vi "Read Analog Waveforms.vi"(8 "error in":errorcluster, 10 "analog task":refnum<k21>) -> (0 "error out":errorcluster, 2 "analog task out":refnum<k21>, 3 "waveforms":waveform(dbl)[](array[waveform]))   [LabVIEW 2021]
uses:
  <vilib>/DAQmx/read.llb/DAQmx Read (Analog 1D Wfm NChan NSamp).vi
  <vilib>/DAQmx/miscellaneous.llb/DAQmx Fill In Error Info.vi
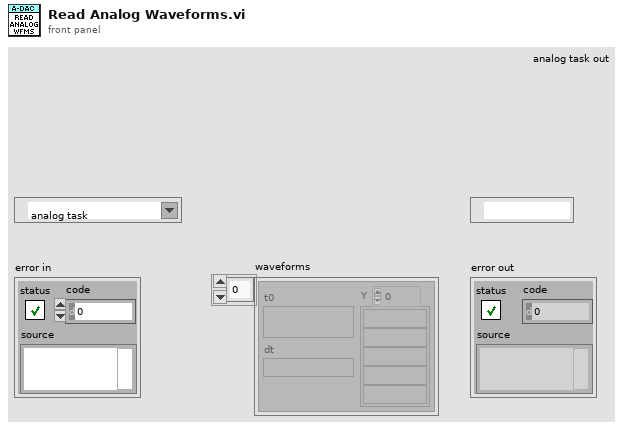
[diagram p1: front panel]
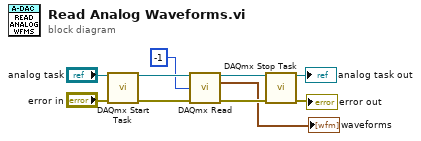
[diagram p0: block diagram]
diagram:
  n1 = call <vilib>:"DAQmx Start Task.vi"("task/channels in"="analog task", "error in"="error in") -> ("task out"=w8:refnum<k21>, "error out"=w10:errorcluster)  [unwired: 12 in]
  n2 = call-poly <vilib>:"DAQmx Read.vi"("task/channels in"=w8, "number of samples per channel"=-1, "error in"=w10) -> ("task out"=w7:refnum<k21>, "data"=→"waveforms":waveform(dbl)[], "error out"=w9:errorcluster)  [unwired: 10 in]
  n3 = call <vilib>:"DAQmx Stop Task.vi"("task/channels in"=w7, "error in"=w9) -> ("task out"=→"analog task out":refnum<k21>, "error out"=→"error out":errorcluster)  [unwired: 12 in]
